vi "get autopop.vi"(8 "error in":errorcluster, 11 "ProjectItem in":refnum<vi>) -> (0 "error out":errorcluster, 1 "private":path[](array[path]), 2 "public":path[](array[path]), 3 "ProjectItem out":refnum<vi>)   [LabVIEW 2013]
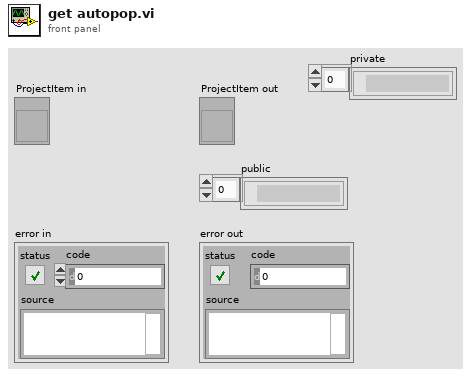
[diagram p1: front panel]
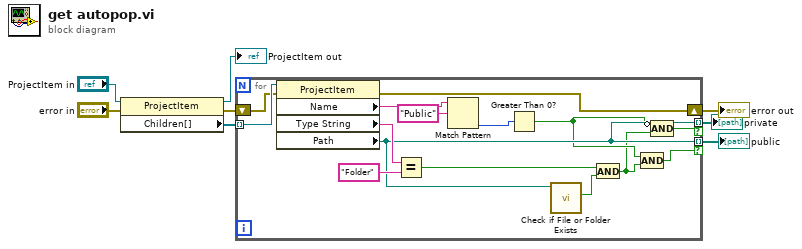
[diagram p0: block diagram]
diagram:
  n1 = property class="ProjectItem"(reference="ProjectItem in", error in="error in") -> (reference out=→"ProjectItem out":refnum<vi>, error out=w3:errorcluster, "Children[]"=w4:refnum<vi>[])
  n2 = for {
    shift-right: [w18] -> w5
    shift-left: w3 -> [w22]
    tunnel: w4 -> [w23] mode=indexing
    tunnel: [w14] -> w6 mode=indexing if=w12
    tunnel: [w14] -> w1 mode=indexing if=w10
    n3 = property class="ProjectItem"(reference=w23, error in=w22) -> (error out=w18:errorcluster, "Name"=w16:string, "Type String"=w21:string, "Path"=w14:path)  [unwired: 1 out]
    n4 = Equal?(x=w21, y="Folder") -> (x = y?=w19:bool)
    n5 = Match Pattern(string=w16, regular expression="Public") -> (offset past match=w13:i32)  [unwired: 1 in, 3 out]
    n6 = Greater Than 0?(x=w13) -> (x > 0?=w11:bool)
    n7 = call <vilib>:"Check if File or Folder Exists.vi"("path"=w14) -> ("file or folder exists?"=w17:bool)  [unwired: 8 in, 2 out]
    n8 = And(x=w19, y=w17) -> (x .and. y?=w9:bool)
    n9 = Compound Arithmetic op=AND(w11, w9) -> (w12:bool)
    n10 = Compound Arithmetic op=AND(invert w11, w9) -> (w10:bool)
  }
  "public" <- w6
  "error out" <- w5
  "private" <- w1
